vi "make_plot_data_mesh_color_ramp.vi"(4 "Absolute Color mapping":bool, 6 "Interpolate Color":bool, 8 "Amplitude":T1, 9 "Number of Colors":i32, 10 "Alpha":dbl=1.0, 11 "Color Ramp Array":cluster{dbl, u32}[](array[cluster])) -> (2 "Array":u32[](array[numeric]), 3 "Color Array":cluster{"R":sgl, "G":sgl, "B":sgl, "A":sgl}[](array[cluster]))   [LabVIEW 2020, in "3DPC_SurfacePlot.xctl"]
uses:
  <vilib>/Native 3D Graph/xcontrol/3DPC_SurfacePlot.xctl
  <vilib>/Native 3D Graph/typedefs/min_max.ctl
  <vilib>/picture/3D Picture Control/NI_3D Picture Control.lvlib
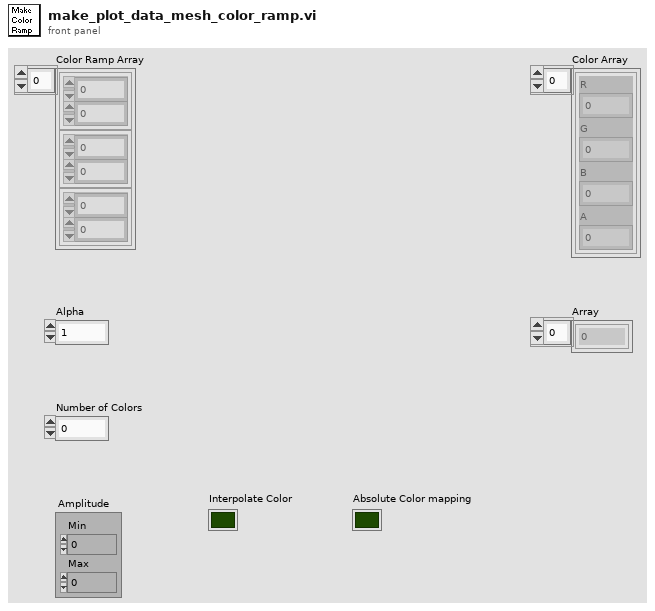
[diagram p1: front panel]
types:
  T1 = typedef "3DPC_SurfacePlot.xctl/min_max.ctl" = cluster{"Min":sgl, "Max":sgl}
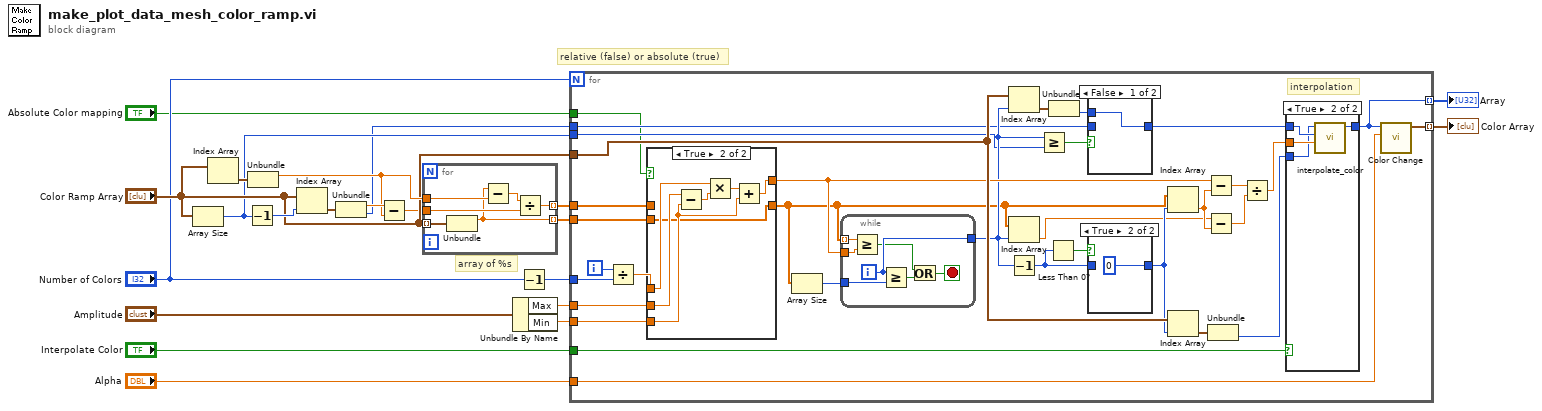
[diagram p0: block diagram]
diagram:
  # "relative (false) or absolute (true)"
  # "array of %s"
  n1 = Array Size(array="Color Ramp Array") -> (size(s)=w12:i32)
  n2 = Index Array(array="Color Ramp Array") -> (element=w20:cluster{dbl, u32})  [unwired: 1 in]
  n3 = Decrement(x=w12) -> (x-1=w21:i32)
  n4 = Unbundle(w20) -> (w17:dbl)  [unwired: 1 out]
  n5 = Index Array(array="Color Ramp Array", index=w21) -> (element=w19:cluster{dbl, u32})
  n6 = Unbundle(w19) -> (w18:dbl, w11:u32)
  n7 = Subtract(x=w18, y=w17) -> (x-y=w14:dbl)
  n8 = for {
    tunnel: w14 -> [w26]
    tunnel: "Color Ramp Array" -> [w27] mode=indexing
    tunnel: [w25] -> w13 mode=indexing
    tunnel: w17 -> [w24]
    tunnel: [w22] -> w8 mode=indexing
    n9 = Unbundle(w27) -> (w22:dbl)  [unwired: 1 out]
    n10 = Subtract(x=w22, y=w24) -> (x-y=w23:dbl)
    n11 = Divide(x=w23, y=w26) -> (x/y=w25:dbl)
  }
  n12 = Unbundle By Name("Amplitude") -> ("Max"=w1:sgl, "Min"=w7:sgl)
  n13 = Decrement(x="Number of Colors") -> (x-1=w10:i32)
  n14 = for {
    N: "Number of Colors" -> [_]
    tunnel: w13 -> [w34]
    tunnel: "Color Ramp Array" -> [w55]
    tunnel: [w49] -> w6 mode=indexing
    tunnel: w7 -> [w48]
    tunnel: w1 -> [w47]
    tunnel: w12 -> [w40]
    tunnel: w11 -> [w37]
    tunnel: w10 -> [w35]
    tunnel: w8 -> [w32]
    tunnel: [w31] -> w5 mode=indexing
    tunnel: "Alpha" -> [w30]
    tunnel: "Interpolate Color" -> [w29]
    tunnel: "Absolute Color mapping" -> [w28]
    i -> [w60]
    # "interpolation"
    n15 = Divide(x=w60, y=w35) -> (x/y=w46:dbl)
    n16 = case shown="True" w28 {
      tunnel: w48 -> [_ w73]
      tunnel: w47 -> [_ w76]
      tunnel: w46 -> [w69 w75]
      tunnel: [w69 w71] -> w43
      tunnel: w34 -> [w68 _]
      tunnel: [w68 w70] -> w33
      tunnel: w32 -> [_ w70]
      frame False {
      }
      frame True {
        n17 = Subtract(x=w76, y=w73) -> (x-y=w74:sgl)
        n18 = Multiply(x=w75, y=w74) -> (x*y=w72:dbl)
        n19 = Add(x=w72, y=w73) -> (x+y=w71:dbl)
      }
    }
    n20 = Array Size(array=w33) -> (size(s)=w59:i32)
    n21 = while {
      tunnel: w33 -> [w81] mode=indexing
      tunnel: w43 -> [w80]
      tunnel: w59 -> [w85]
      tunnel: [w82] -> w41
      i -> [w82]
      stop <- w83 stop-if-true
      n22 = Greater Or Equal?(x=w81, y=w80) -> (x >= y?=w79:bool)
      n23 = Greater Or Equal?(x=w82, y=w85) -> (x >= y?=w84:bool)
      n24 = Or(x=w79, y=w84) -> (x .or. y?=w83:bool)
    }
    n25 = Index Array(array=w55, index=w41) -> (element=w53:cluster{dbl, u32})
    n26 = Index Array(array=w33, index=w41) -> (element=w42:dbl)
    n27 = Decrement(x=w41) -> (x-1=w50:i32)
    n28 = Greater Or Equal?(x=w41, y=w40) -> (x >= y?=w39:bool)
    n29 = Less Than 0?(x=w50) -> (x < 0?=w52:bool)
    n30 = Unbundle(w53) -> (w38:u32)  [unwired: 1 out]
    n31 = case shown="False" w39 {
      tunnel: w38 -> [w61 _]
      tunnel: w37 -> [_ w62]
      tunnel: [w61 w62] -> w36
      frame False {
      }
      frame True {
      }
    }
    n32 = case shown="True" w52 {
      tunnel: [w77 0 ("index")] -> w51
      tunnel: w50 -> [w77 _]
      frame False {
      }
      frame True {
      }
    }
    n33 = Index Array(array=w33, index=w51) -> (element=w58:dbl)
    n34 = Index Array(array=w55, index=w51) -> (element=w54:cluster{dbl, u32})
    n35 = Subtract(x=w43, y=w58) -> (x-y=w44:dbl)
    n36 = Subtract(x=w42, y=w58) -> (x-y=w57:dbl)
    n37 = Unbundle(w54) -> (w45:u32)  [unwired: 1 out]
    n38 = Divide(x=w44, y=w57) -> (x/y=w56:dbl)
    n39 = case shown="True" w29 {
      tunnel: w56 -> [_ w67]
      tunnel: w36 -> [_ w66]
      tunnel: [w63 w65] -> w49
      tunnel: w45 -> [w63 w64]
      frame False {
      }
      frame True {
        n40 = call <vilib>:"interpolate_color.vi"("Interpolation Value"=w67, "Color2"=w66, "Color1"=w64) -> ("Output Color"=w65:u32)  [unwired: 8 out]
      }
    }
    n41 = call <vilib>:"Color Change.vi"("Alpha"=w30, "Color"=w49) -> ("RGBA"=w31:cluster{"R":sgl, "G":sgl, "B":sgl, "A":sgl})  [unwired: 9 out]
  }
  "Color Array" <- w5
  "Array" <- w6
